vi "XIPIN_SMPTE2022-5_6_Video_over_IP_Receiver_2_1.vi"   [LabVIEW 2017]
doc: "The Xilinx LogiCORE IP SMPTE2022-5/6 Video over IP Receiver is a module for broadcast applications that requires bridging between SMPTE video connectivity standards (SD/HD/ 3G-SDI) and 10Gb/s networks. The module is capable of recovering IP packets lost to network transmission errors and ensure the picture quality of uncompressed, high bandwidth professional video.\n------------------------------------\n<b>Need License</b> : Yes\n<b>Interface</b> : AXI4 AXI4-Stream AXI4-Lite"
uses:
  <vilib>/rvi/XilinxIP/XIPIN_XNode/niFpgaXIPIN.xnode
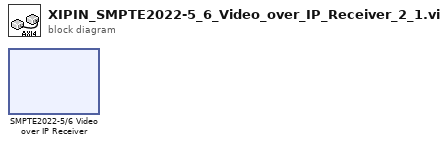
[diagram p0: block diagram]
diagram:
  n1 = xnode ("SMPTE2022-5/6 Video over IP Receiver")() -> ()
